vi "Index VI.vi"(6 "DBMap":refnum<class "DBMap.lvclass">, 7 "VI to analyze":path=path "C:/Projects/DMC/VISight/Source/Analyzer/Fibonacci.vi", 8 "error in (no error)":errorcluster, 9 "Valid Terminals Set":set{string}(c389)={"ControlTerminal", "OverridableParameterTerminal", "Terminal"}, 10 "AtomicSet":refnum<class "DBSet.lvclass">) -> (0 "error out":errorcluster, 3 "Node to children":T1(c390))   [LabVIEW 2024]
uses:
  <vilib>/Utility/miscctls.llb/LVMapReplaceAction.ctl
  DBSet/DBSet.lvclass
  DBMap/DBMap.lvclass
  <vilib>/Utility/traverseref.llb/VI Scripting - Traverse.lvlib
  <vilib>/Utility/traverseref.llb/TRef TravTarget.ctl
  <vilib>/security/Message Digest/API/NI_Message Digest API.lvlib
  <vilib>/security/Message Digest/API/Instances/File/SHA-256 File Checksum.vi
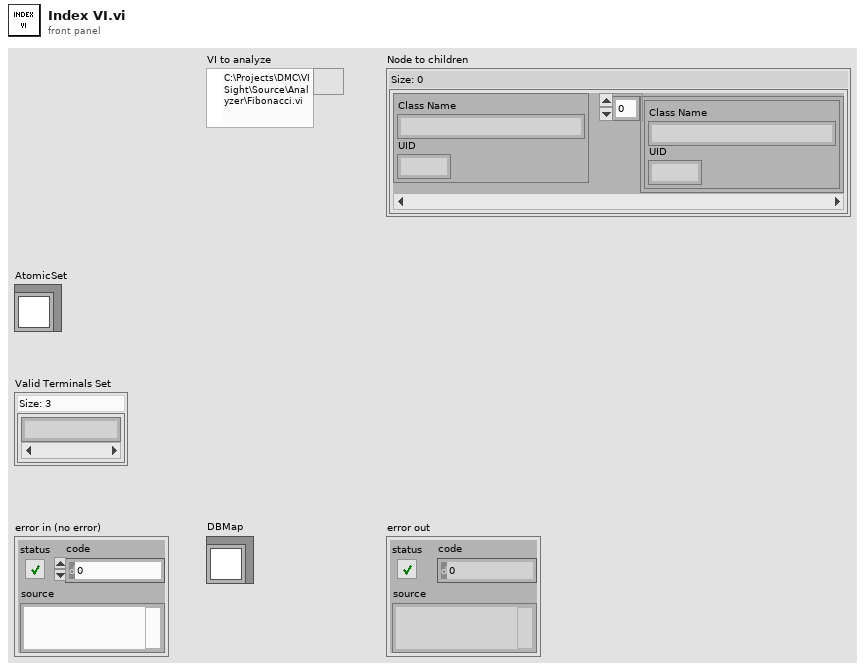
[diagram p1: front panel]
types:
  T1 = map{cluster{"Class Name":string, "UID":i32}, cluster{"Class Name":string, "UID":i32}[]}
  T2 = typedef "TRef TravTarget.ctl" = enum16{"FP", "BD", "Other"}
  T3 = typedef "LVMapReplaceAction.ctl" = enum32{"Modify Entry only if found", "Add or Modify Entry", "Delete Entry"}
  T4 = cluster{"ClassName":string, "Caption":string, "UID":i32}
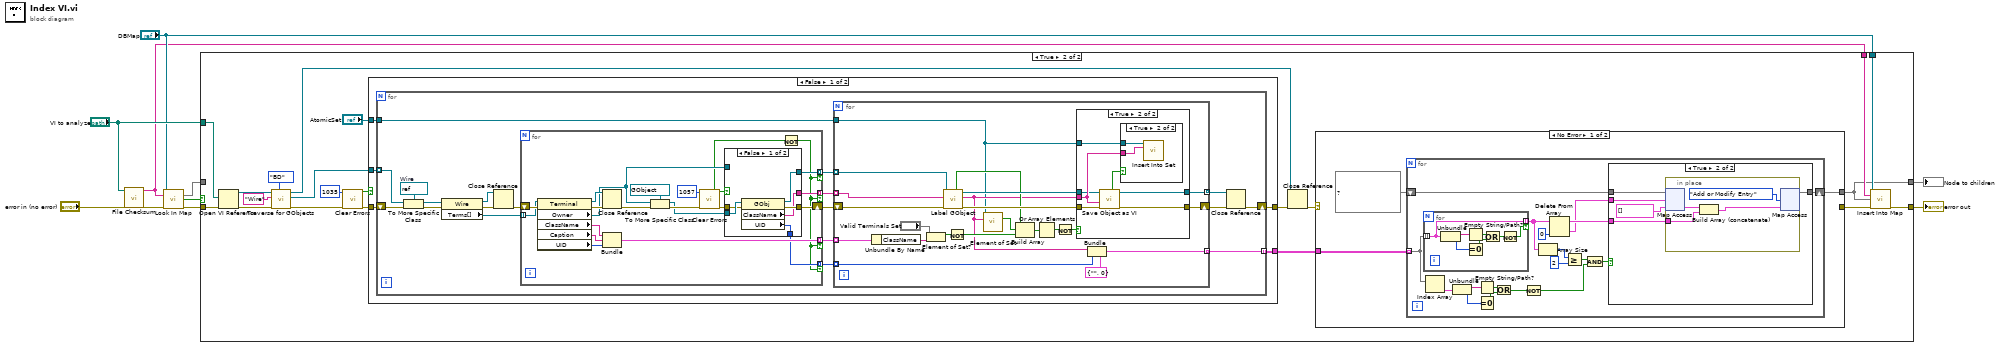
[diagram p0: block diagram]
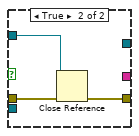
[diagram p5: hidden frame]
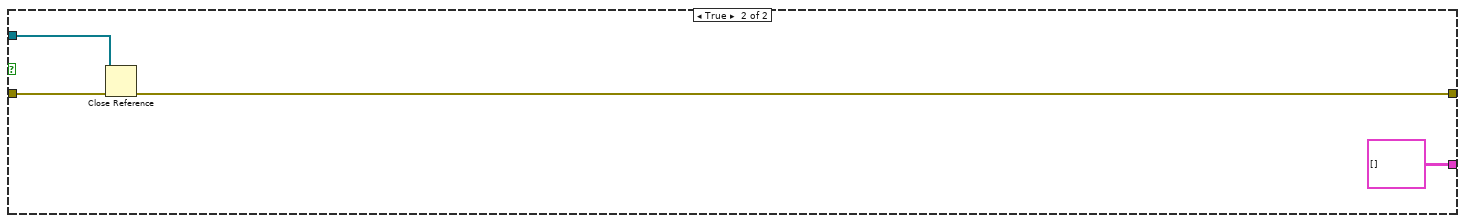
[diagram p6: hidden frame]
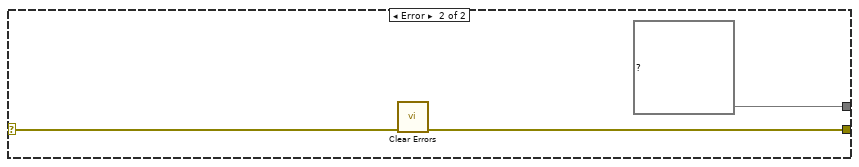
[diagram p8: hidden frame]
diagram:
  n1 = call-poly <vilib>:"File Checksum.vi"("path"="VI to analyze") -> ("digest"=w2:string)  [unwired: 9 in, 1 out]
  n2 = call "Look In Map.vi"("DBMap in"="DBMap", "Key"=w2, "error in (no error)"="error in (no error)") -> ("Map"=w4:T1, "Not Found?"=w1:bool, "error out"=w5:errorcluster)  [unwired: 9 in, 1 out]
  n3 = case shown="True" w1 {
    tunnel: [w11 w20] -> w9
    tunnel: [w10 w22] -> w8
    tunnel: "VI to analyze" -> [_ w25]
    tunnel: w5 -> [w10 w19]
    tunnel: w4 -> [w11 _]
    tunnel: "DBMap" -> [_ w24]
    tunnel: w2 -> [_ w21]
    frame False {
    }
    frame True {
      n4 = Open VI Reference(vi path=w25, error in (no error)=w19) -> (vi reference=w15:refnum<vi>, error out=w16:errorcluster)  [unwired: 4 in]
      n5 = call <vilib>:"Traverse for GObjects.vi"("Traverse Target"=TRef_TravTarget."BD", "error in (no error)"=w16, "Class Name"="Wire", "VI Refnum"=w15) -> ("error out"=w13:errorcluster, "References"=w12:refnum<vi>[], "dup VI Refnum"=w14:refnum<vi>)  [unwired: 4 in, 1 out]
      n6 = call <vilib>:"Clear Errors.vi"("error in (no error)"=w13, "specific error code to clear (0: all)"=1035) -> ("error out"=w30:errorcluster, "specific error cleared?"=w28:bool)  [unwired: 4 in]
      n7 = case shown="False" w28 {
        tunnel: [w36 w122] -> w32
        tunnel: [w35 cluster{"Class Name":string, "UID":i32}[][] []] -> w31
        tunnel: w30 -> [w34 w121]
        tunnel: w12 -> [w37 w123]
        tunnel: "AtomicSet" -> [w33 _]
        frame False {
          n8 = for {
            tunnel: w37 -> [w39] mode=indexing
            shift-right: [w43] -> w36
            shift-left: w34 -> [w42]
            tunnel: [w49] -> w35 mode=indexing
            tunnel: w33 -> [w44]
            w38 = refnum<vi> refnum  # Wire
            n9 = To More Specific Class(target class=w38, reference=w39, error in=w42) -> (specific class reference=w40:refnum<vi>, error out=w41:errorcluster)
            n10 = property on="Property Node" class="Wire"(reference=w40, error in=w41) -> (reference out=w46:refnum<vi>, error out=w48:errorcluster, "Terms[]"=w56:refnum<vi>[])
            n11 = Close Reference(reference=w46, error in (no error)=w48) -> (error out=w47:errorcluster)
            n12 = for {
              tunnel: [w92] -> w53 mode=indexing if=w90
              tunnel: [w94] -> w52 mode=indexing if=w90
              shift-right: [w93] -> w51
              shift-left: w47 -> [w110]
              tunnel: w56 -> [w108] mode=indexing
              tunnel: [w91] -> w50 mode=indexing if=w90
              tunnel: [w104] -> w54 mode=indexing if=w90
              n13 = property on="Property Node" class="Terminal"(reference=w108, error in=w110) -> (reference out=w103:refnum<vi>, error out=w102:errorcluster, "Owner"=w98:refnum<vi>, "ClassName"=w107:string, "Caption"=w106:string, "UID"=w105:i32)
              n14 = Close Reference(reference=w103, error in (no error)=w102) -> (error out=w101:errorcluster)
              n15 = Bundle("ClassName"=w107, "Caption"=w106, "UID"=w105) -> (w104:T4)  [unwired: 1 in]
              n16 = To More Specific Class(target class=refnum<vi> refnum ("reference"), reference=w98, error in=w101) -> (specific class reference=w95:refnum<vi>, error out=w100:errorcluster)
              n17 = call <vilib>:"Clear Errors.vi"("error in (no error)"=w100, "specific error code to clear (0: all)"=1057) -> ("error out"=w97:errorcluster, "specific error cleared?"=w96:bool)  [unwired: 4 in]
              n18 = case shown="False" w96 {
                tunnel: w98 -> [_ w118]
                tunnel: w97 -> [w115 w119]
                tunnel: w95 -> [w116 _]
                tunnel: [w114 _] -> w94
                tunnel: [w113 w117] -> w93
                tunnel: [w112 _] -> w92
                tunnel: [w111 _] -> w91
                frame False {
                  n19 = property class="GObj"(reference=w116, error in=w115) -> (reference out=w114:refnum<vi>, error out=w113:errorcluster, "ClassName"=w112:string, "UID"=w111:i32)
                }
                frame True {
                  n20 = Close Reference(reference=w118, error in (no error)=w119) -> (error out=w117:errorcluster)
                }
              }
              n21 = Not(x=w96) -> (.not. x?=w90:bool)
            }
            n22 = for {
              tunnel: w52 -> [w62] mode=indexing
              tunnel: w53 -> [w63] mode=indexing
              shift-right: [w74] -> w55
              shift-left: w51 -> [w65]
              tunnel: [w73] -> w45 mode=indexing
              tunnel: w54 -> [w78] mode=indexing
              tunnel: w50 -> [w76] mode=indexing
              tunnel: [w75] -> w49 mode=indexing
              tunnel: w44 -> [w57]
              n23 = Unbundle By Name(w78) -> ("ClassName"=w72:string)
              n24 = Element of Set?(10:w72, 11:"Valid Terminals Set") -> (3:w77:bool)
              n25 = call "Label GObject.vi"("error in"=w65, "GObject ClassName"=w63, "GObject Reference In"=w62) -> ("error out"=w64:errorcluster, "Label"=w59:string, "GObject Reference out"=w61:refnum<vi>, "Excluded?"=w60:bool)  [unwired: 4 in, 1 out]
              n26 = Not(x=w77) -> (.not. x?=w68:bool)
              n27 = call "Element of Set.vi"("DBSet in"=w57, "Element"=w59) -> ("Found?"=w58:bool)  [unwired: 11 in, 2 out]
              n28 = Build Array(w60, w58, w68) -> (w67:bool[])
              n29 = Or Array Elements(Boolean array=w67) -> (logical OR=w66:bool)
              n30 = Not(x=w66) -> (.not. x?=w69:bool)
              n31 = case shown="True" w69 {
                tunnel: w61 -> [w79 w83]
                tunnel: w59 -> [_ w87]
                tunnel: w64 -> [w80 w86]
                tunnel: [w80 w85] -> w74
                tunnel: [w79 w84] -> w73
                tunnel: w57 -> [_ w81]
                frame False {
                }
                frame True {
                  n32 = call "Save Object as VI.vi"("error in (no error)"=w86, "Name"=w87, "Object in"=w83) -> ("error out"=w85:errorcluster, "Object out"=w84:refnum<vi>, "Ok?"=w82:bool)  [unwired: 6 in]
                  n33 = case shown="True" w82 {
                    tunnel: w87 -> [_ w88]
                    tunnel: w81 -> [_ w89]
                    frame False {
                    }
                    frame True {
                      n34 = call "Insert Into Set.vi"("DBSet in"=w89, "Element"=w88) -> ()  [unwired: 12 in, 2 out]
                    }
                  }
                }
              }
              n35 = Bundle(cluster=cluster{"Class Name":string, "UID":i32} {"Class Name"="", "UID"=0} ("Source"), "Class Name"=w59, "UID"=w76) -> (w75:cluster{"Class Name":string, "UID":i32})
            }
            n36 = Close Reference(reference=w45, error in (no error)=w55) -> (error out=w43:errorcluster)
          }
        }
        frame True {
          n37 = Close Reference(reference=w123, error in (no error)=w121) -> (error out=w122:errorcluster)
        }
      }
      n38 = Close Reference(reference=w14, error in (no error)=w32) -> (error out=w27:errorcluster)
      n39 = case shown="No Error" w27 {
        selector: w27 -> [_ w164]
        tunnel: w31 -> [w126 _]
        tunnel: [w124 T1 {} ("map in")] -> w20
        tunnel: [_ w162] -> w23
        frame No Error {
          n40 = for {
            tunnel: w126 -> [w136] mode=indexing
            shift-right: [w127] -> w124
            shift-left: T1 {} ("map in") -> [w132]
            n41 = for {
              tunnel: w136 -> [w157] mode=indexing
              tunnel: [w157] -> w130 mode=indexing if=w155
              n42 = Unbundle(w157) -> ("Class Name"=w158:string, "UID"=w159:i32)
              n43 = Empty String/Path?(string/path=w158) -> (empty?=w160:bool)
              n44 = Equal To 0?(x=w159) -> (x = 0?=w161:bool)
              n45 = Or(x=w160, y=w161) -> (x .or. y?=w156:bool)
              n46 = Not(x=w156) -> (.not. x?=w155:bool)
            }
            n47 = Index Array(array=w136) -> (element=w139:cluster{"Class Name":string, "UID":i32})  [unwired: 1 in]
            n48 = Unbundle(w139) -> ("Class Name"=w144:string, "UID"=w143:i32)
            n49 = Empty String/Path?(string/path=w144) -> (empty?=w142:bool)
            n50 = Equal To 0?(x=w143) -> (x = 0?=w141:bool)
            n51 = Or(x=w142, y=w141) -> (x .or. y?=w140:bool)
            n52 = Not(x=w140) -> (.not. x?=w134:bool)
            n53 = Array Size(array=w130) -> (size(s)=w138:i32)
            n54 = Delete From Array(array=w130, index=0) -> (deleted portion=w128:cluster{"Class Name":string, "UID":i32}, array with subset deleted=w129:cluster{"Class Name":string, "UID":i32}[])  [unwired: 1 in]
            n55 = Greater Or Equal?(x=w138, y=2) -> (x >= y?=w135:bool)
            n56 = And(x=w135, y=w134) -> (x .and. y?=w133:bool)
            n57 = case shown="True" w133 {
              tunnel: w132 -> [w145 w149]
              tunnel: w129 -> [_ w146]
              tunnel: w128 -> [_ w147]
              tunnel: [w145 w148] -> w127
              frame False {
              }
              frame True {
                n58 = in-place {
                  in-place-border: w146 -> [w151]
                  n59 = in-place-map #1(w149, w147, cluster{"Class Name":string, "UID":i32}[] [] ("value")) -> (w154:cluster{"Class Name":string, "UID":i32}[])  [unwired: 1 out]
                  n60 = Build Array (concatenate)(w154, w151) -> (w153:cluster{"Class Name":string, "UID":i32}[])
                  n61 = in-place-map #1(w153, LVMapReplaceAction."Add or Modify Entry" ("action")) -> (w148:T1)  [unwired: 2 out]
                }
              }
            }
          }
        }
        frame Error {
          n62 = call <vilib>:"Clear Errors.vi"("error in (no error)"=w164) -> ("error out"=w162:errorcluster)  [unwired: 5 in, 1 out]
        }
      }
      n63 = call "Insert Into Map.vi"("DBMap in"=w24, "Key"=w21, "Value"=w20, "error in (no error)"=w23) -> ("error out"=w22:errorcluster)  [unwired: 10 in, 1 out]
    }
  }
  "error out" <- w8
  "Node to children" <- w9
